vi "Constants.vi"() -> ()   [LabVIEW 2015, in "Host Heartbeat Shared.lvlib"]
doc: "Use this Global VI to access the GUIDs assigned to the page resources of the Custom Device."
uses:
  Host Heartbeat Shared.lvlib
panel:
  in  "Tab Control":enum32{"GUIDS", "Constants", "Properties"}(tab)
  in  "Host Heartbeat":string="8fa418f6-73f5-4d4c-ae4c-b43013d0febf"
  in  "TCP Daemon Port":string="TCPDaemonPort"
  in  "TCP Remote Port":string="TCPRemotePort"
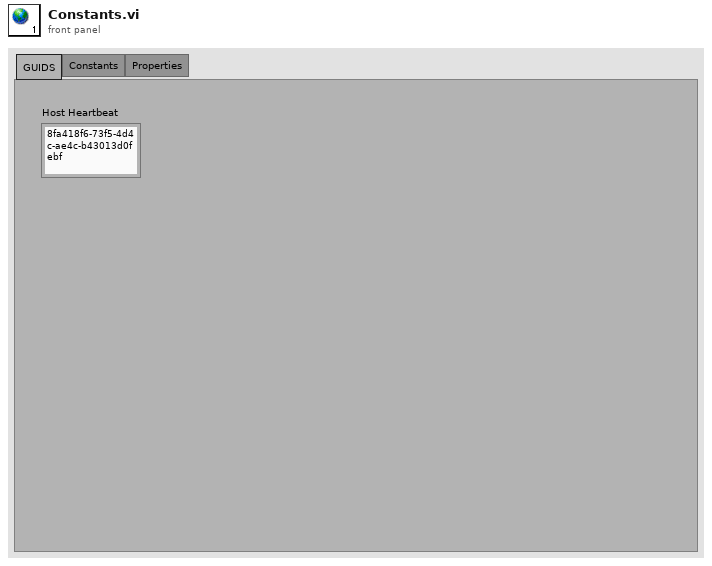
[diagram p1: front panel]
diagram:
